vi "Read_XML_Parameters File_002.vi"(8 "error in (no error)":errorcluster, 11 "XML Configuration File Path":path=path "C:/Users/Vincent/Desktop/Ballard-Arinc-429-Custom-Device Inline Async/Testing/Parameters Configuration File/XML_Parameters_002_B.xml") -> (0 "error out":errorcluster, 3 "Channels":T1[](array[typedef]))   [LabVIEW 2019, in "Ballard Arinc-429 System Explorer.lvlib"]
uses:
  Ballard Arinc-429 System Explorer.lvlib
  XML_Channel.ctl
  XML_Label.ctl
  XML_Parameter.ctl
  C:/Users/Localization Tester/Desktop/GIT/Ballard-Arinc-429-Custom-Device/Source/System Explorer/SubVIs/Parse Parameters File/Parameters_Arinc429_XML_Tools.dll
  Parameters_Arinc429_XML_Tools.dll
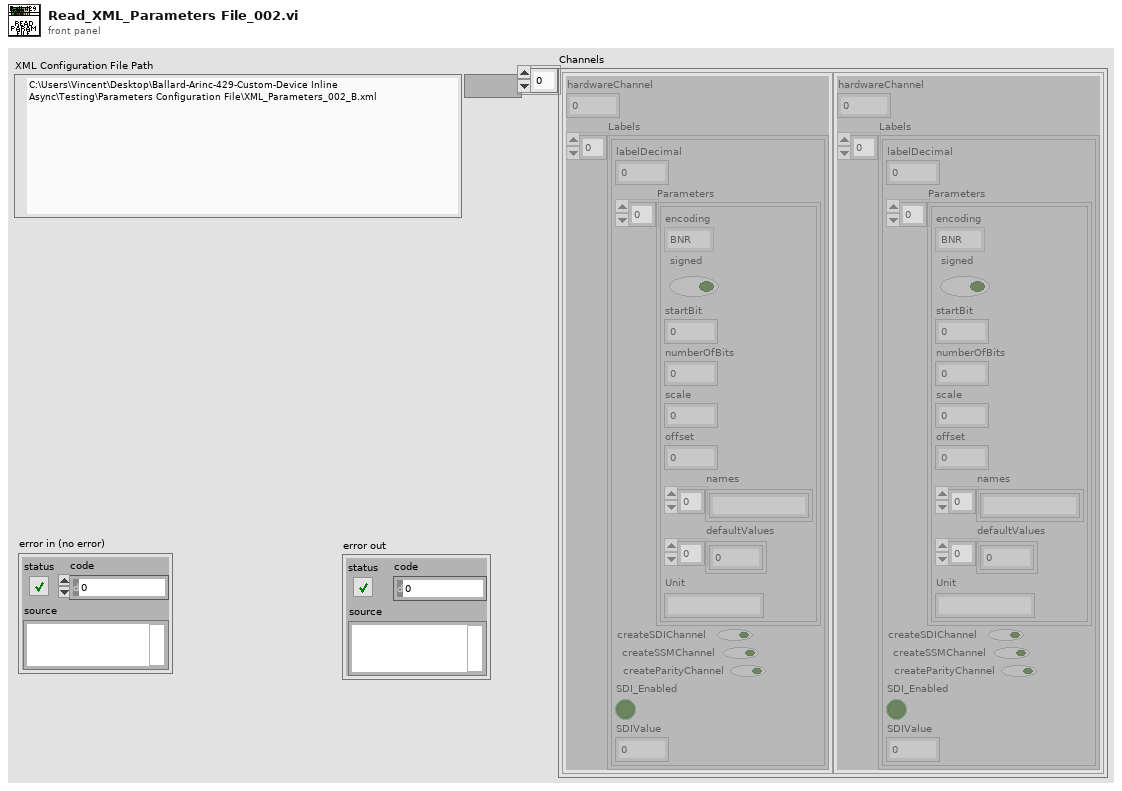
[diagram p1: front panel]
types:
  T1 = typedef "XML_Channel.ctl" = cluster{"hardwareChannel":i32, "Labels":T2[]}
  T2 = typedef "XML_Label.ctl" = cluster{"labelDecimal":i32, "Parameters":T3[], "createSDIChannel":bool, "createSSMChannel":bool, "createParityChannel":bool, "SDI_Enabled":bool, "SDIValue":u8}
  T3 = typedef "XML_Parameter.ctl" = cluster{"encoding":enum16{"BNR", "BCD", "Discrete"}, "signed":bool, "startBit":i32, "numberOfBits":i32, "scale":dbl, "offset":dbl, "names":string[], "defaultValues":dbl[], "Unit":string}
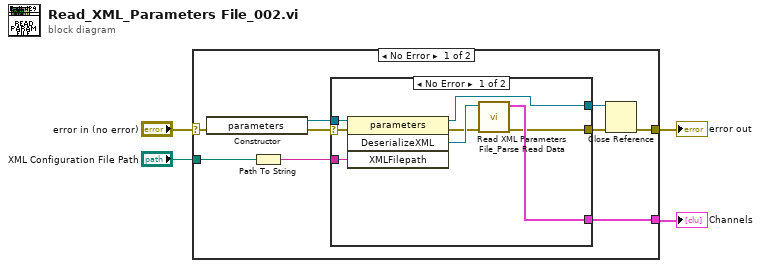
[diagram p0: block diagram]
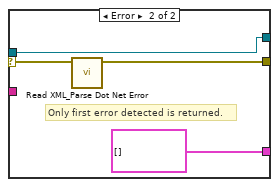
[diagram p2: hidden frame]
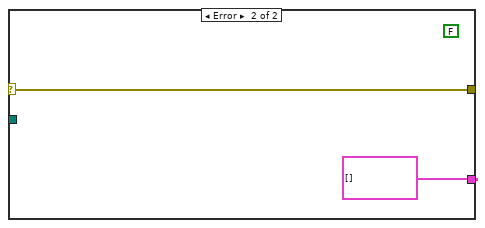
[diagram p3: hidden frame]
diagram:
  n1 = case shown="No Error" "error in (no error)" {
    selector: "error in (no error)" -> [w11 w27]
    tunnel: "XML Configuration File Path" -> [w13 _]
    tunnel: [w5 w27] -> w3
    tunnel: [w10 T1[] [] ("Channels")] -> w1
    frame No Error {
      n2 = constructor class="parameters"(error in=w11) -> (reference out=w8:refnum<k24>, error out=w9:errorcluster)  [unwired: 2 in, 1 out]
      n3 = Path To String(path=w13) -> (string=w12:string)
      n4 = case shown="No Error" w9 {
        selector: w9 -> [w16 w25]
        tunnel: [w14 w24] -> w7
        tunnel: w12 -> [w21 _]
        tunnel: w8 -> [w17 w22]
        tunnel: [w18 T1[] [] ("Channels")] -> w10
        tunnel: [w15 w22] -> w6
        frame No Error {
          n5 = invoke class="parameters" method="DeserializeXML"(reference=w17, error in=w16, "XMLFilepath"=w21) -> (reference out=w15:refnum<k24>, error out=w19:errorcluster, "DeserializeXML"=w20:refnum<k24>)  [unwired: 1 in, 1 out]
          n6 = call "Read XML Parameters File_Parse Read Data.vi"("error in (no error)"=w19, ".NET Refnum in"=w20) -> ("error out"=w14:errorcluster, "Channels"=w18:T1[])  [unwired: 7 in, 1 out]
        }
        frame Error {
          # "Only first error detected is returned."
          n7 = call "Read XML_Parse Dot Net Error.vi"("error in (no error)"=w25) -> ("error out"=w24:errorcluster)  [unwired: 10 in]
        }
      }
      n8 = Close Reference(reference=w6, error in (no error)=w7) -> (error out=w5:errorcluster)
    }
    frame Error {
      (unwired) FALSE ("ValidateAgainstXMLSchema")
    }
  }
  "error out" <- w3
  "Channels" <- w1
